vi "test_CCDGetDataSize.vi"(7 "Test should pass":bool=TRUE, 8 "error in":errorcluster, 9 "tear down connection":bool=TRUE, 10 "set-up a connection":bool=TRUE, 11 "device selection":enum16{"monochromator", "CCD", "SCD"}(ring)=enum."CCD") -> (0 "error out":errorcluster)   [LabVIEW 2023]
uses:
  <vilib>/addons/_JKI Toolkits/Caraya/classes/Test/Test.lvclass
  <vilib>/addons/_JKI Toolkits/Caraya/classes/Assert/Assert.lvclass
  <vilib>/addons/_JKI Toolkits/Caraya/classes/Assert/Assert Not Error.vi
  <vilib>/addons/_JKI Toolkits/Caraya/classes/Assert/Assert Equal Value and Type_Variant.vi
  Classes/CCD/CCD.lvclass
panel:
  # "Connector Pane"
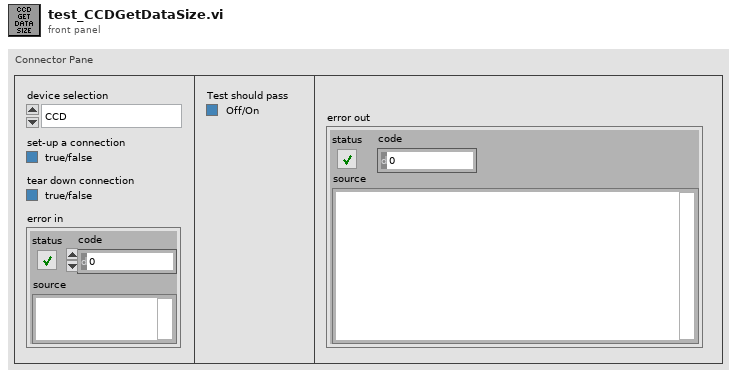
[diagram p1: front panel]
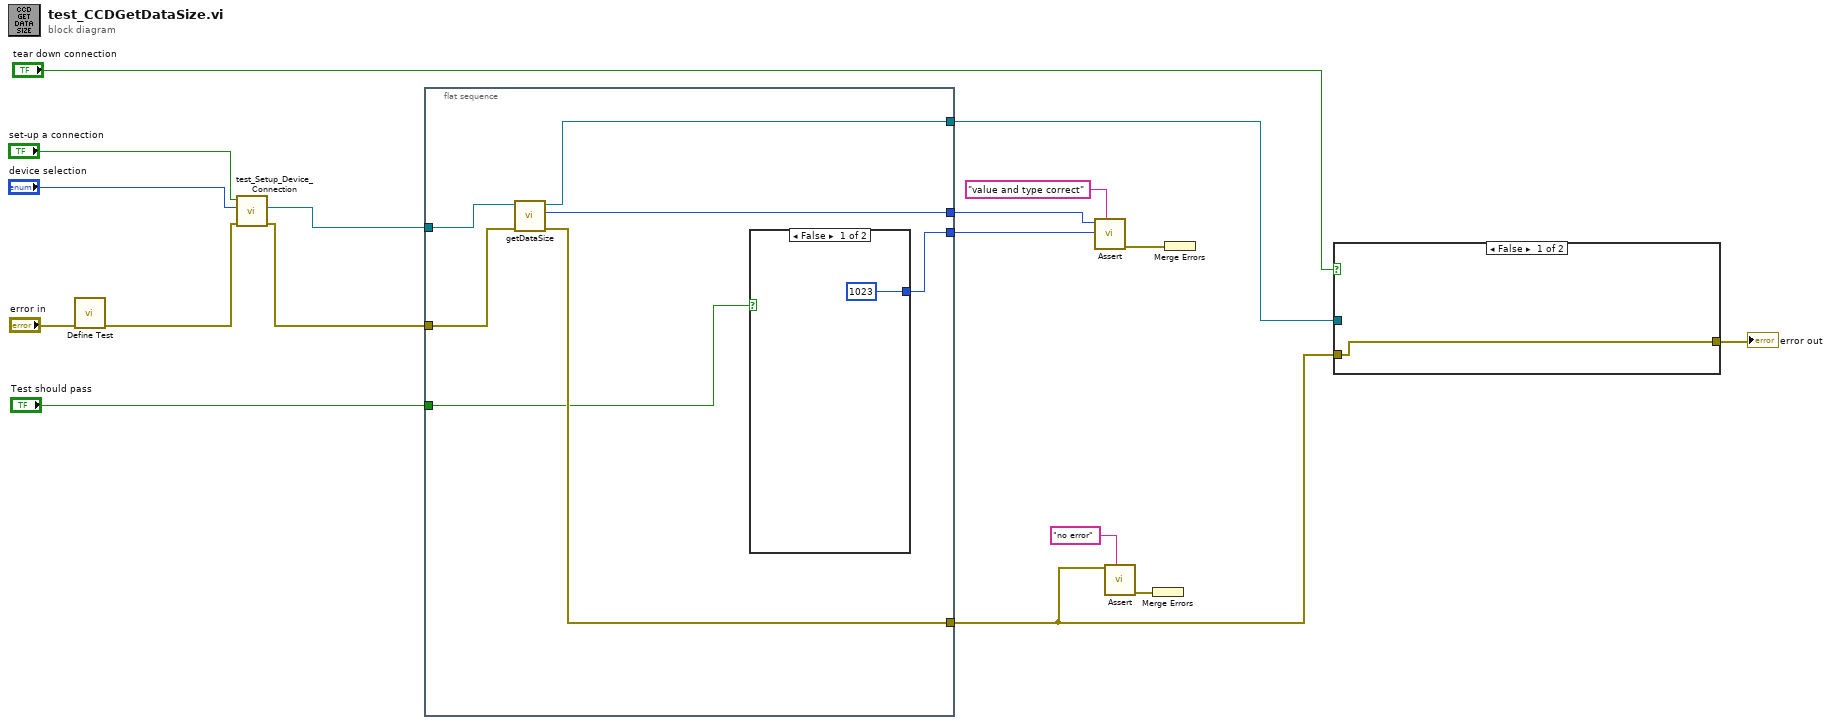
[diagram p0: block diagram]
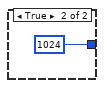
[diagram p2: hidden frame]
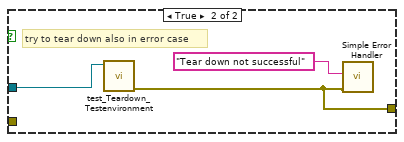
[diagram p3: hidden frame]
diagram:
  n1 = call <vilib>:"Define Test.vi"("error in (no error)"="error in") -> ("error out"=w1:errorcluster)  [unwired: 9 in, 1 out]
  n2 = call "test_Setup_Device_Connection.vi"("error in (no error)"=w1, "device selection"="device selection", "set-up a connection"="set-up a connection") -> ("error out"=w2:errorcluster, "CCD out"=w3:refnum<class "CCD.lvclass">)  [unwired: 5 in, 2 out]
  n3 = flat-sequence {
    tunnel: [w21] -> w15
    tunnel: w2 -> [w24]
    tunnel: w3 -> [w23]
    tunnel: [w20] -> w13
    tunnel: [w22] -> w8
    tunnel: "Test should pass" -> [w19]
    tunnel: [w18] -> w7
    frame #0 {
      n4 = call "getDataSize.vi"("error in (no error)"=w24, "CCD in"=w23) -> ("error out"=w22:errorcluster, "size"=w21:i32, "CCD out"=w18:refnum<class "CCD.lvclass">)  [unwired: 7 in]
      n5 = case shown="False" w19 {
        tunnel: [1023 1024] -> w20
        frame False {
        }
        frame True {
        }
      }
    }
  }
  n6 = call-poly <vilib>:"Assert.vi"("Label"="value and type correct" ("Label (VI Title)"), "Y"=w13, "X"=w15) -> ("error out"=w16:errorcluster)  [unwired: 7 in, 1 out]
  n7 = call-poly <vilib>:"Assert.vi"("Label"="no error" ("Label (VI Title)"), "Not Error?"=w8) -> ("error out"=w10:errorcluster)  [unwired: 8 in, 1 out]
  n8 = Merge Errors(w10) -> ()  [unwired: 1 out]
  n9 = Merge Errors(w16) -> ()  [unwired: 1 out]
  n10 = case shown="False" "tear down connection" {
    tunnel: w7 -> [_ w29]
    tunnel: [w27 w28] -> w6
    tunnel: w8 -> [w27 _]
    frame False {
    }
    frame True {
      # "try to tear down also in error case"
      n11 = call "test_Teardown_Testenvironment.vi"("GenericDevice.lvclass"=w29) -> ("error out"=w28:errorcluster)  [unwired: 9 in, 1 out]
      n12 = call <vilib>:"Simple Error Handler.vi"("error source (\" \")"="Tear down not successful" ("error source (\" \")"), "error in (no error)"=w28) -> ()  [unwired: 3 in, 5 out]
    }
  }
  "error out" <- w6
